vi "Slope.vi"(0 "Y":dbl, 1 "X":dbl, 2 "XY":dbl, 3 "X2":dbl, 4 "N":dbl, 7 "Y2":dbl) -> (5 "Slope":dbl)   [LabVIEW 2012]
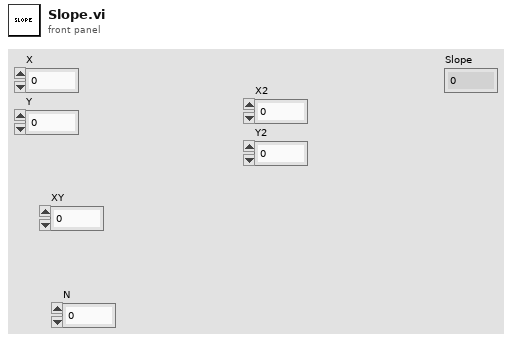
[diagram p1: front panel]
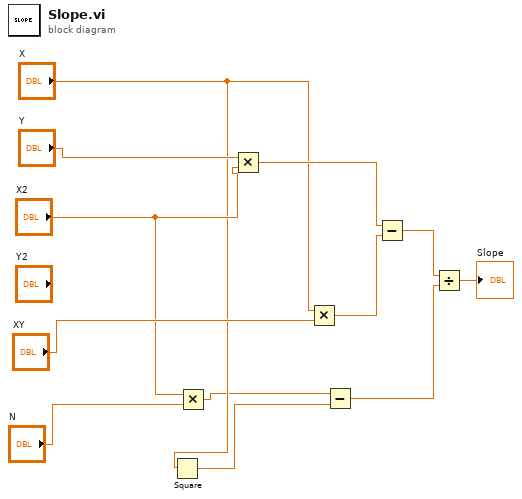
[diagram p0: block diagram]
diagram:
  n1 = Square(x="X") -> (x^2=w5:dbl)
  n2 = Multiply(x="X2", y="N") -> (x*y=w4:dbl)
  n3 = Multiply(x="Y", y="X2") -> (x*y=w11:dbl)
  n4 = Multiply(x="X", y="XY") -> (x*y=w9:dbl)
  n5 = Subtract(x=w4, y=w5) -> (x-y=w2:dbl)
  n6 = Subtract(x=w11, y=w9) -> (x-y=w3:dbl)
  n7 = Divide(x=w3, y=w2) -> (x/y=→"Slope":dbl)
